vi "Main.vi"(7 "sweep rate, /min":dbl=0.2, 8 "sweep to:":dbl=4.0, 9 "sweep":T8(radio)=enum."2636a_smub") -> ()   [LabVIEW 2021] (continued)
                    n2908 = Concatenate Strings(w3787, w3783, "\t") -> (w3786:string)
                  }
                }
                n2909 = property on="Figure_axis" class="Arr (strict)"("Value"=w3775) -> ()  [unwired: 2 in, 2 out]
                n2910 = property on="data_caption" class="Str"("Value"=w3777) -> ()  [unwired: 2 in, 2 out]
              }
              frame #11 {
                # "2400 1 current measure (2400_1_i)"
                n2911 = local read "2400 1 meas i"() -> (w3794:bool)
                n2912 = property on="Figure_axis" class="Arr (strict)"() -> ("Value"=w3791:string[])  [unwired: 2 in, 2 out]
                n2913 = property on="data_caption" class="Str"() -> ("Value"=w3793:string)  [unwired: 2 in, 2 out]
                n2914 = case shown="False" w3794 {
                  tunnel: w3793 -> [w3796 w3802]
                  tunnel: [w3796 w3801] -> w3792
                  tunnel: w3791 -> [w3795 w3799]
                  tunnel: [w3795 w3797] -> w3790
                  frame False {
                    # "not measure 2400 1 current (2400_1_i)"
                  }
                  frame True {
                    w3798 = "2400_1_i"
                    # "measure 2400 1 current (2400_1_i)"
                    n2915 = local read "2400 1 addr"() -> (w3803:u8)
                    n2916 = Number To Decimal String(number=w3803) -> (decimal integer string=w3804:string)  [unwired: 1 in]
                    n2917 = GPIB Clear(3:w3804) -> ()  [unwired: 1 in, 2 out]
                    n2918 = Build Array (concatenate)(w3799, w3798) -> (w3797:string[])
                    n2919 = Concatenate Strings(w3802, w3798, "\t") -> (w3801:string)
                  }
                }
                n2920 = property on="Figure_axis" class="Arr (strict)"("Value"=w3790) -> ()  [unwired: 2 in, 2 out]
                n2921 = property on="data_caption" class="Str"("Value"=w3792) -> ()  [unwired: 2 in, 2 out]
              }
              frame #12 {
                # "2400 2 voltage measure (2400_2_v)"
                n2922 = local read "2400 2 meas v"() -> (w3809:bool)
                n2923 = property on="Figure_axis" class="Arr (strict)"() -> ("Value"=w3806:string[])  [unwired: 2 in, 2 out]
                n2924 = property on="data_caption" class="Str"() -> ("Value"=w3808:string)  [unwired: 2 in, 2 out]
                n2925 = case shown="False" w3809 {
                  tunnel: w3808 -> [w3811 w3817]
                  tunnel: [w3811 w3816] -> w3807
                  tunnel: w3806 -> [w3810 w3814]
                  tunnel: [w3810 w3812] -> w3805
                  frame False {
                    # "not measure 2400 2 voltage (2400_2_v)"
                  }
                  frame True {
                    w3813 = "2400_2_v"
                    # "measure 2400 2 voltage (2400_2_v)"
                    n2926 = local read "2400 2 addr"() -> (w3818:u8)
                    n2927 = Number To Decimal String(number=w3818) -> (decimal integer string=w3819:string)  [unwired: 1 in]
                    n2928 = GPIB Clear(3:w3819) -> ()  [unwired: 1 in, 2 out]
                    n2929 = Build Array (concatenate)(w3814, w3813) -> (w3812:string[])
                    n2930 = Concatenate Strings(w3817, w3813, "\t") -> (w3816:string)
                  }
                }
                n2931 = property on="Figure_axis" class="Arr (strict)"("Value"=w3805) -> ()  [unwired: 2 in, 2 out]
                n2932 = property on="data_caption" class="Str"("Value"=w3807) -> ()  [unwired: 2 in, 2 out]
              }
              frame #13 {
                # "2400 2 current measure (2400_2_i)"
                n2933 = local read "2400 2 meas i"() -> (w3824:bool)
                n2934 = property on="Figure_axis" class="Arr (strict)"() -> ("Value"=w3821:string[])  [unwired: 2 in, 2 out]
                n2935 = property on="data_caption" class="Str"() -> ("Value"=w3823:string)  [unwired: 2 in, 2 out]
                n2936 = case shown="False" w3824 {
                  tunnel: w3823 -> [w3826 w3832]
                  tunnel: [w3826 w3831] -> w3822
                  tunnel: w3821 -> [w3825 w3829]
                  tunnel: [w3825 w3827] -> w3820
                  frame False {
                    # "not measure 2400 2 current (2400_2_i)"
                  }
                  frame True {
                    w3828 = "2400_2_i"
                    # "measure 2400 2 current (2400_2_i)"
                    n2937 = local read "2400 2 addr"() -> (w3833:u8)
                    n2938 = Number To Decimal String(number=w3833) -> (decimal integer string=w3834:string)  [unwired: 1 in]
                    n2939 = GPIB Clear(3:w3834) -> ()  [unwired: 1 in, 2 out]
                    n2940 = Build Array (concatenate)(w3829, w3828) -> (w3827:string[])
                    n2941 = Concatenate Strings(w3832, w3828, "\t") -> (w3831:string)
                  }
                }
                n2942 = property on="Figure_axis" class="Arr (strict)"("Value"=w3820) -> ()  [unwired: 2 in, 2 out]
                n2943 = property on="data_caption" class="Str"("Value"=w3822) -> ()  [unwired: 2 in, 2 out]
              }
              frame #14 {
                # "2400 3 voltage measure (2400_3_v)"
                n2944 = local read "2400 3 meas v"() -> (w3839:bool)
                n2945 = property on="Figure_axis" class="Arr (strict)"() -> ("Value"=w3836:string[])  [unwired: 2 in, 2 out]
                n2946 = property on="data_caption" class="Str"() -> ("Value"=w3838:string)  [unwired: 2 in, 2 out]
                n2947 = case shown="False" w3839 {
                  tunnel: w3838 -> [w3841 w3847]
                  tunnel: [w3841 w3846] -> w3837
                  tunnel: w3836 -> [w3840 w3844]
                  tunnel: [w3840 w3842] -> w3835
                  frame False {
                    # "not measure 2400 3 voltage (2400_3_v)"
                  }
                  frame True {
                    w3843 = "2400_3_v"
                    # "measure 2400 3 voltage (2400_3_v)"
                    n2948 = local read "2400 3 addr"() -> (w3848:u8)
                    n2949 = Number To Decimal String(number=w3848) -> (decimal integer string=w3849:string)  [unwired: 1 in]
                    n2950 = GPIB Clear(3:w3849) -> ()  [unwired: 1 in, 2 out]
                    n2951 = Build Array (concatenate)(w3844, w3843) -> (w3842:string[])
                    n2952 = Concatenate Strings(w3847, w3843, "\t") -> (w3846:string)
                  }
                }
                n2953 = property on="Figure_axis" class="Arr (strict)"("Value"=w3835) -> ()  [unwired: 2 in, 2 out]
                n2954 = property on="data_caption" class="Str"("Value"=w3837) -> ()  [unwired: 2 in, 2 out]
              }
              frame #15 {
                # "2400 3 current measure (2400_3_i)"
                n2955 = local read "2400 3 meas i"() -> (w3854:bool)
                n2956 = property on="Figure_axis" class="Arr (strict)"() -> ("Value"=w3851:string[])  [unwired: 2 in, 2 out]
                n2957 = property on="data_caption" class="Str"() -> ("Value"=w3853:string)  [unwired: 2 in, 2 out]
                n2958 = case shown="True" w3854 {
                  tunnel: w3853 -> [w3856 w3862]
                  tunnel: [w3856 w3861] -> w3852
                  tunnel: w3851 -> [w3855 w3859]
                  tunnel: [w3855 w3857] -> w3850
                  frame False {
                    # "not measure 2400 3 current (2400_3_i)"
                  }
                  frame True {
                    w3858 = "2400_3_i"
                    # "measure 2400 3 current (2400_3_i)"
                    n2959 = local read "2400 3 addr"() -> (w3863:u8)
                    n2960 = Number To Decimal String(number=w3863) -> (decimal integer string=w3864:string)  [unwired: 1 in]
                    n2961 = GPIB Clear(3:w3864) -> ()  [unwired: 1 in, 2 out]
                    n2962 = Build Array (concatenate)(w3859, w3858) -> (w3857:string[])
                    n2963 = Concatenate Strings(w3862, w3858, "\t") -> (w3861:string)
                  }
                }
                n2964 = property on="Figure_axis" class="Arr (strict)"("Value"=w3850) -> ()  [unwired: 2 in, 2 out]
                n2965 = property on="data_caption" class="Str"("Value"=w3852) -> ()  [unwired: 2 in, 2 out]
              }
              frame #16 {
                # "2182A 1 channel 1 measure (2182A_1_ch1)"
                n2966 = local read "2182A 1 ch1"() -> (w3869:bool)
                n2967 = property on="Figure_axis" class="Arr (strict)"() -> ("Value"=w3866:string[])  [unwired: 2 in, 2 out]
                n2968 = property on="data_caption" class="Str"() -> ("Value"=w3868:string)  [unwired: 2 in, 2 out]
                n2969 = case shown="False" w3869 {
                  tunnel: w3868 -> [w3871 w3877]
                  tunnel: [w3871 w3876] -> w3867
                  tunnel: w3866 -> [w3870 w3874]
                  tunnel: [w3870 w3872] -> w3865
                  frame False {
                    # "not measure 2182A 1 channel 1 (2182A_1_ch1)"
                  }
                  frame True {
                    w3873 = "2182A_1_ch1"
                    # "measure 2182A 1 channel 1 (2182A_1_ch1)"
                    n2970 = local read "2182A 1 addr"() -> (w3878:u8)
                    n2971 = Number To Decimal String(number=w3878) -> (decimal integer string=w3879:string)  [unwired: 1 in]
                    n2972 = GPIB Clear(3:w3879) -> ()  [unwired: 1 in, 2 out]
                    n2973 = Build Array (concatenate)(w3874, w3873) -> (w3872:string[])
                    n2974 = Concatenate Strings(w3877, w3873, "\t") -> (w3876:string)
                  }
                }
                n2975 = property on="Figure_axis" class="Arr (strict)"("Value"=w3865) -> ()  [unwired: 2 in, 2 out]
                n2976 = property on="data_caption" class="Str"("Value"=w3867) -> ()  [unwired: 2 in, 2 out]
              }
              frame #17 {
                # "2182A 1 channel 2 measure (2182A_1_ch2)"
                n2977 = local read "2182A 1 ch2"() -> (w3884:bool)
                n2978 = property on="Figure_axis" class="Arr (strict)"() -> ("Value"=w3881:string[])  [unwired: 2 in, 2 out]
                n2979 = property on="data_caption" class="Str"() -> ("Value"=w3883:string)  [unwired: 2 in, 2 out]
                n2980 = case shown="True" w3884 {
                  tunnel: w3883 -> [w3886 w3892]
                  tunnel: [w3886 w3891] -> w3882
                  tunnel: w3881 -> [w3885 w3889]
                  tunnel: [w3885 w3887] -> w3880
                  frame False {
                    # "not measure 2182A 1 channel 2 (2182A_1_ch2)"
                  }
                  frame True {
                    w3888 = "2182A_1_ch2"
                    # "measure 2182A 1 channel 2 (2182A_1_ch2)"
                    n2981 = local read "2182A 1 addr"() -> (w3893:u8)
                    n2982 = Number To Decimal String(number=w3893) -> (decimal integer string=w3894:string)  [unwired: 1 in]
                    n2983 = GPIB Clear(3:w3894) -> ()  [unwired: 1 in, 2 out]
                    n2984 = Build Array (concatenate)(w3889, w3888) -> (w3887:string[])
                    n2985 = Concatenate Strings(w3892, w3888, "\t") -> (w3891:string)
                  }
                }
                n2986 = property on="Figure_axis" class="Arr (strict)"("Value"=w3880) -> ()  [unwired: 2 in, 2 out]
                n2987 = property on="data_caption" class="Str"("Value"=w3882) -> ()  [unwired: 2 in, 2 out]
              }
              frame #18 {
                # "2182A 2 channel 1 measure (2182A_2_ch1)"
                n2988 = local read "2182A 2 ch1"() -> (w3899:bool)
                n2989 = property on="Figure_axis" class="Arr (strict)"() -> ("Value"=w3896:string[])  [unwired: 2 in, 2 out]
                n2990 = property on="data_caption" class="Str"() -> ("Value"=w3898:string)  [unwired: 2 in, 2 out]
                n2991 = case shown="True" w3899 {
                  tunnel: w3898 -> [w3901 w3907]
                  tunnel: [w3901 w3906] -> w3897
                  tunnel: w3896 -> [w3900 w3904]
                  tunnel: [w3900 w3902] -> w3895
                  frame False {
                    # "not measure 2182A 2 channel 1 (2182A_2_ch1)"
                  }
                  frame True {
                    w3903 = "2182A_2_ch1"
                    # "measure 2182A 2 channel 1 (2182A_2_ch1)"
                    n2992 = local read "2182A 2 addr"() -> (w3908:u8)
                    n2993 = Number To Decimal String(number=w3908) -> (decimal integer string=w3909:string)  [unwired: 1 in]
                    n2994 = GPIB Clear(3:w3909) -> ()  [unwired: 1 in, 2 out]
                    n2995 = Build Array (concatenate)(w3904, w3903) -> (w3902:string[])
                    n2996 = Concatenate Strings(w3907, w3903, "\t") -> (w3906:string)
                  }
                }
                n2997 = property on="Figure_axis" class="Arr (strict)"("Value"=w3895) -> ()  [unwired: 2 in, 2 out]
                n2998 = property on="data_caption" class="Str"("Value"=w3897) -> ()  [unwired: 2 in, 2 out]
              }
              frame #19 {
                # "2182A 2 channel 2 measure (2182A_2_ch2)"
                n2999 = local read "2182A 2 ch2"() -> (w3914:bool)
                n3000 = property on="Figure_axis" class="Arr (strict)"() -> ("Value"=w3911:string[])  [unwired: 2 in, 2 out]
                n3001 = property on="data_caption" class="Str"() -> ("Value"=w3913:string)  [unwired: 2 in, 2 out]
                n3002 = case shown="True" w3914 {
                  tunnel: w3913 -> [w3916 w3922]
                  tunnel: [w3916 w3921] -> w3912
                  tunnel: w3911 -> [w3915 w3919]
                  tunnel: [w3915 w3917] -> w3910
                  frame False {
                    # "not measure 2182A 2 channel 2 (2182A_2_ch2)"
                  }
                  frame True {
                    w3918 = "2182A_2_ch2"
                    # "measure 2182A 2 channel 2 (2182A_2_ch2)"
                    n3003 = local read "2182A 2 addr"() -> (w3923:u8)
                    n3004 = Number To Decimal String(number=w3923) -> (decimal integer string=w3924:string)  [unwired: 1 in]
                    n3005 = GPIB Clear(3:w3924) -> ()  [unwired: 1 in, 2 out]
                    n3006 = Build Array (concatenate)(w3919, w3918) -> (w3917:string[])
                    n3007 = Concatenate Strings(w3922, w3918, "\t") -> (w3921:string)
                  }
                }
                n3008 = property on="Figure_axis" class="Arr (strict)"("Value"=w3910) -> ()  [unwired: 2 in, 2 out]
                n3009 = property on="data_caption" class="Str"("Value"=w3912) -> ()  [unwired: 2 in, 2 out]
              }
              frame #20 {
                # "2182A 3 channel 1 measure (2182A_3_ch1)"
                n3010 = local read "2182A 3 ch1"() -> (w3929:bool)
                n3011 = property on="Figure_axis" class="Arr (strict)"() -> ("Value"=w3926:string[])  [unwired: 2 in, 2 out]
                n3012 = property on="data_caption" class="Str"() -> ("Value"=w3928:string)  [unwired: 2 in, 2 out]
                n3013 = case shown="True" w3929 {
                  tunnel: w3928 -> [w3931 w3937]
                  tunnel: [w3931 w3936] -> w3927
                  tunnel: w3926 -> [w3930 w3934]
                  tunnel: [w3930 w3932] -> w3925
                  frame False {
                    # "not measure 2182A 3 channel 1 (2182A_3_ch1)"
                  }
                  frame True {
                    w3933 = "2182A_3_ch1"
                    # "measure 2182A 3 channel 1 (2182A_3_ch1)"
                    n3014 = local read "2182A 3 addr"() -> (w3938:u8)
                    n3015 = Number To Decimal String(number=w3938) -> (decimal integer string=w3939:string)  [unwired: 1 in]
                    n3016 = GPIB Clear(3:w3939) -> ()  [unwired: 1 in, 2 out]
                    n3017 = Build Array (concatenate)(w3934, w3933) -> (w3932:string[])
                    n3018 = Concatenate Strings(w3937, w3933, "\t") -> (w3936:string)
                  }
                }
                n3019 = property on="Figure_axis" class="Arr (strict)"("Value"=w3925) -> ()  [unwired: 2 in, 2 out]
                n3020 = property on="data_caption" class="Str"("Value"=w3927) -> ()  [unwired: 2 in, 2 out]
              }
              frame #21 {
                # "2182A 3 channel 2 measure (2182A_3_ch2)"
                n3021 = local read "2182A 3 ch2"() -> (w3944:bool)
                n3022 = property on="Figure_axis" class="Arr (strict)"() -> ("Value"=w3941:string[])  [unwired: 2 in, 2 out]
                n3023 = property on="data_caption" class="Str"() -> ("Value"=w3943:string)  [unwired: 2 in, 2 out]
                n3024 = case shown="False" w3944 {
                  tunnel: w3943 -> [w3946 w3952]
                  tunnel: [w3946 w3951] -> w3942
                  tunnel: w3941 -> [w3945 w3949]
                  tunnel: [w3945 w3947] -> w3940
                  frame False {
                    # "not measure 2182A 3 channel 2 (2182A_3_ch2)"
                  }
                  frame True {
                    w3948 = "2182A_3_ch2"
                    # "measure 2182A 3 channel 2 (2182A_3_ch2)"
                    n3025 = local read "2182A 3 addr"() -> (w3953:u8)
                    n3026 = Number To Decimal String(number=w3953) -> (decimal integer string=w3954:string)  [unwired: 1 in]
                    n3027 = GPIB Clear(3:w3954) -> ()  [unwired: 1 in, 2 out]
                    n3028 = Build Array (concatenate)(w3949, w3948) -> (w3947:string[])
                    n3029 = Concatenate Strings(w3952, w3948, "\t") -> (w3951:string)
                  }
                }
                n3030 = property on="Figure_axis" class="Arr (strict)"("Value"=w3940) -> ()  [unwired: 2 in, 2 out]
                n3031 = property on="data_caption" class="Str"("Value"=w3942) -> ()  [unwired: 2 in, 2 out]
              }
              frame #22 {
                # "2182A 4 channel 1 measure (2182A_4_ch1)"
                n3032 = local read "2182A 4 ch1"() -> (w3959:bool)
                n3033 = property on="Figure_axis" class="Arr (strict)"() -> ("Value"=w3956:string[])  [unwired: 2 in, 2 out]
                n3034 = property on="data_caption" class="Str"() -> ("Value"=w3958:string)  [unwired: 2 in, 2 out]
                n3035 = case shown="True" w3959 {
                  tunnel: w3958 -> [w3961 w3967]
                  tunnel: [w3961 w3966] -> w3957
                  tunnel: w3956 -> [w3960 w3964]
                  tunnel: [w3960 w3962] -> w3955
                  frame False {
                    # "not measure 2182A 4 channel 1 (2182A_4_ch1)"
                  }
                  frame True {
                    w3963 = "2182A_4_ch1"
                    # "measure 2182A 4 channel 1 (2182A_4_ch1)"
                    n3036 = local read "2182A 4 addr"() -> (w3968:u8)
                    n3037 = Number To Decimal String(number=w3968) -> (decimal integer string=w3969:string)  [unwired: 1 in]
                    n3038 = GPIB Clear(3:w3969) -> ()  [unwired: 1 in, 2 out]
                    n3039 = Build Array (concatenate)(w3964, w3963) -> (w3962:string[])
                    n3040 = Concatenate Strings(w3967, w3963, "\t") -> (w3966:string)
                  }
                }
                n3041 = property on="Figure_axis" class="Arr (strict)"("Value"=w3955) -> ()  [unwired: 2 in, 2 out]
                n3042 = property on="data_caption" class="Str"("Value"=w3957) -> ()  [unwired: 2 in, 2 out]
              }
              frame #23 {
                # "2182A 4 channel 2 measure (2182A_4_ch2)"
                n3043 = local read "2182A 4 ch2"() -> (w3974:bool)
                n3044 = property on="Figure_axis" class="Arr (strict)"() -> ("Value"=w3971:string[])  [unwired: 2 in, 2 out]
                n3045 = property on="data_caption" class="Str"() -> ("Value"=w3973:string)  [unwired: 2 in, 2 out]
                n3046 = case shown="True" w3974 {
                  tunnel: w3973 -> [w3976 w3982]
                  tunnel: [w3976 w3981] -> w3972
                  tunnel: w3971 -> [w3975 w3979]
                  tunnel: [w3975 w3977] -> w3970
                  frame False {
                    # "not measure 2182A 4 channel 2 (2182A_4_ch2)"
                  }
                  frame True {
                    w3978 = "2182A_4_ch2"
                    # "measure 2182A 4 channel 2 (2182A_4_ch2)"
                    n3047 = local read "2182A 4 addr"() -> (w3983:u8)
                    n3048 = Number To Decimal String(number=w3983) -> (decimal integer string=w3984:string)  [unwired: 1 in]
                    n3049 = GPIB Clear(3:w3984) -> ()  [unwired: 1 in, 2 out]
                    n3050 = Build Array (concatenate)(w3979, w3978) -> (w3977:string[])
                    n3051 = Concatenate Strings(w3982, w3978, "\t") -> (w3981:string)
                  }
                }
                n3052 = property on="Figure_axis" class="Arr (strict)"("Value"=w3970) -> ()  [unwired: 2 in, 2 out]
                n3053 = property on="data_caption" class="Str"("Value"=w3972) -> ()  [unwired: 2 in, 2 out]
              }
              frame #24 {
                # "2636A smua measure voltage (2636A_smua_v)"
                n3054 = local read "2636A smua meas v"() -> (w3989:bool)
                n3055 = property on="Figure_axis" class="Arr (strict)"() -> ("Value"=w3986:string[])  [unwired: 2 in, 2 out]
                n3056 = property on="data_caption" class="Str"() -> ("Value"=w3988:string)  [unwired: 2 in, 2 out]
                n3057 = case shown="True" w3989 {
                  tunnel: w3988 -> [w3991 w4002]
                  tunnel: [w3991 w4001] -> w3987
                  tunnel: w3986 -> [w3990 w3999]
                  tunnel: [w3990 w3997] -> w3985
                  frame False {
                    # "not measure voltage on 2636A smua (2636A_smua_v)"
                  }
                  frame True {
                    w3998 = "2636A_smua_v"
                    # "measure voltage on 2636A smua (2636A_smua_v)"
                    n3058 = local read "2614A addr"() -> (w3993:refnum<visa-resource-name>)
                    n3059 = VISA Open(VISA resource name=w3993) -> (VISA resource name=w3992:refnum<visa-resource-name>, error out=w3994:errorcluster)  [unwired: 4 in]
                    n3060 = VISA Clear(VISA resource name=w3992, error in (no error)=w3994) -> (VISA resource name out=w3996:refnum<visa-resource-name>)  [unwired: 1 out]
                    n3061 = property class="Instr"(reference=w3996, "General Settings:Timeout Value"=u32 10000) -> ()  [unwired: 1 in, 2 out]
                    n3062 = Build Array (concatenate)(w3999, w3998) -> (w3997:string[])
                    n3063 = Concatenate Strings(w4002, w3998, "\t") -> (w4001:string)
                  }
                }
                n3064 = property on="Figure_axis" class="Arr (strict)"("Value"=w3985) -> ()  [unwired: 2 in, 2 out]
                n3065 = property on="data_caption" class="Str"("Value"=w3987) -> ()  [unwired: 2 in, 2 out]
              }
              frame #25 {
                # "2636A smua measure current (2636A_smua_i)"
                n3066 = local read "2636A smua meas i"() -> (w4007:bool)
                n3067 = property on="Figure_axis" class="Arr (strict)"() -> ("Value"=w4004:string[])  [unwired: 2 in, 2 out]
                n3068 = property on="data_caption" class="Str"() -> ("Value"=w4006:string)  [unwired: 2 in, 2 out]
                n3069 = case shown="True" w4007 {
                  tunnel: w4006 -> [w4009 w4020]
                  tunnel: [w4009 w4019] -> w4005
                  tunnel: w4004 -> [w4008 w4017]
                  tunnel: [w4008 w4015] -> w4003
                  frame False {
                    # "not measure current on 2636A smua (2636A_smua_i)"
                  }
                  frame True {
                    w4016 = "2636A_smua_i"
                    # "measure current on 2636A smua (2636A_smua_i)"
                    n3070 = local read "2614A addr"() -> (w4012:refnum<visa-resource-name>)
                    n3071 = VISA Open(VISA resource name=w4012) -> (VISA resource name=w4011:refnum<visa-resource-name>, error out=w4010:errorcluster)  [unwired: 4 in]
                    n3072 = VISA Clear(VISA resource name=w4011, error in (no error)=w4010) -> (VISA resource name out=w4013:refnum<visa-resource-name>)  [unwired: 1 out]
                    n3073 = Build Array (concatenate)(w4017, w4016) -> (w4015:string[])
                    n3074 = property class="Instr"(reference=w4013, "General Settings:Timeout Value"=u32 10000) -> ()  [unwired: 1 in, 2 out]
                    n3075 = Concatenate Strings(w4020, w4016, "\t") -> (w4019:string)
                  }
                }
                n3076 = property on="Figure_axis" class="Arr (strict)"("Value"=w4003) -> ()  [unwired: 2 in, 2 out]
                n3077 = property on="data_caption" class="Str"("Value"=w4005) -> ()  [unwired: 2 in, 2 out]
              }
              frame #26 {
                # "2636A smub measure voltage (2636A_smub_v)"
                n3078 = local read "2636A smub meas v"() -> (w4025:bool)
                n3079 = property on="Figure_axis" class="Arr (strict)"() -> ("Value"=w4022:string[])  [unwired: 2 in, 2 out]
                n3080 = property on="data_caption" class="Str"() -> ("Value"=w4024:string)  [unwired: 2 in, 2 out]
                n3081 = case shown="True" w4025 {
                  tunnel: w4024 -> [w4027 w4038]
                  tunnel: [w4027 w4037] -> w4023
                  tunnel: w4022 -> [w4026 w4035]
                  tunnel: [w4026 w4033] -> w4021
                  frame False {
                    # "not measure voltage on 2636A smub (2636A_smub_v)"
                  }
                  frame True {
                    w4034 = "2636A_smub_v"
                    # "measure voltage on 2636A smub (2636A_smub_v)"
                    n3082 = local read "2614A addr"() -> (w4029:refnum<visa-resource-name>)
                    n3083 = VISA Open(VISA resource name=w4029) -> (VISA resource name=w4028:refnum<visa-resource-name>, error out=w4030:errorcluster)  [unwired: 4 in]
                    n3084 = VISA Clear(VISA resource name=w4028, error in (no error)=w4030) -> (VISA resource name out=w4031:refnum<visa-resource-name>)  [unwired: 1 out]
                    n3085 = Build Array (concatenate)(w4035, w4034) -> (w4033:string[])
                    n3086 = property class="Instr"(reference=w4031, "General Settings:Timeout Value"=u32 10000) -> ()  [unwired: 1 in, 2 out]
                    n3087 = Concatenate Strings(w4038, w4034, "\t") -> (w4037:string)
                  }
                }
                n3088 = property on="Figure_axis" class="Arr (strict)"("Value"=w4021) -> ()  [unwired: 2 in, 2 out]
                n3089 = property on="data_caption" class="Str"("Value"=w4023) -> ()  [unwired: 2 in, 2 out]
              }
              frame #27 {
                # "2636A smub measure current (2636A_smub_i)"
                n3090 = local read "2636A smub meas i"() -> (w4043:bool)
                n3091 = property on="Figure_axis" class="Arr (strict)"() -> ("Value"=w4040:string[])  [unwired: 2 in, 2 out]
                n3092 = property on="data_caption" class="Str"() -> ("Value"=w4042:string)  [unwired: 2 in, 2 out]
                n3093 = case shown="True" w4043 {
                  tunnel: w4042 -> [w4045 w4056]
                  tunnel: [w4045 w4055] -> w4041
                  tunnel: w4040 -> [w4044 w4053]
                  tunnel: [w4044 w4051] -> w4039
                  frame False {
                    # "not measure current on 2636A smub (2636A_smub_i)"
                  }
                  frame True {
                    w4052 = "2636A_smub_i"
                    # "measure current on 2636A smub (2636A_smub_i)"
                    n3094 = local read "2614A addr"() -> (w4046:refnum<visa-resource-name>)
                    n3095 = VISA Open(VISA resource name=w4046) -> (VISA resource name=w4047:refnum<visa-resource-name>, error out=w4048:errorcluster)  [unwired: 4 in]
                    n3096 = VISA Clear(VISA resource name=w4047, error in (no error)=w4048) -> (VISA resource name out=w4049:refnum<visa-resource-name>)  [unwired: 1 out]
                    n3097 = Build Array (concatenate)(w4053, w4052) -> (w4051:string[])
                    n3098 = property class="Instr"(reference=w4049, "General Settings:Timeout Value"=u32 10000) -> ()  [unwired: 1 in, 2 out]
                    n3099 = Concatenate Strings(w4056, w4052, "\t") -> (w4055:string)
                  }
                }
                n3100 = property on="Figure_axis" class="Arr (strict)"("Value"=w4039) -> ()  [unwired: 2 in, 2 out]
                n3101 = property on="data_caption" class="Str"("Value"=w4041) -> ()  [unwired: 2 in, 2 out]
              }
              frame #28 {
                # "measure time"
                n3102 = local read "measure time"() -> (w4061:bool)
                n3103 = property on="Figure_axis" class="Arr (strict)"() -> ("Value"=w4058:string[])  [unwired: 2 in, 2 out]
                n3104 = property on="data_caption" class="Str"() -> ("Value"=w4060:string)  [unwired: 2 in, 2 out]
                n3105 = case shown="True" w4061 {
                  tunnel: w4060 -> [w4063 w4069]
                  tunnel: [w4063 w4068] -> w4059
                  tunnel: w4058 -> [w4062 w4066]
                  tunnel: [w4062 w4064] -> w4057
                  frame False {
                    # "not measuring time"
                  }
                  frame True {
                    w4065 = "time"
                    # "measuring time"
                    n3106 = Build Array (concatenate)(w4066, w4065) -> (w4064:string[])
                    n3107 = Concatenate Strings(w4069, w4065, "\t") -> (w4068:string)
                  }
                }
                n3108 = property on="Figure_axis" class="Arr (strict)"("Value"=w4057) -> ()  [unwired: 2 in, 2 out]
                n3109 = property on="data_caption" class="Str"("Value"=w4059) -> ()  [unwired: 2 in, 2 out]
              }
              frame #29 {
                # "Measure magnetic field on IPS120-0"
                n3110 = local read "MagnetField"() -> (w4074:bool)
                n3111 = property on="Figure_axis" class="Arr (strict)"() -> ("Value"=w4071:string[])  [unwired: 2 in, 2 out]
                n3112 = property on="data_caption" class="Str"() -> ("Value"=w4073:string)  [unwired: 2 in, 2 out]
                n3113 = case shown="True" w4074 {
                  tunnel: w4073 -> [w4076 w4082]
                  tunnel: [w4076 w4081] -> w4072
                  tunnel: w4071 -> [w4075 w4079]
                  tunnel: [w4075 w4077] -> w4070
                  frame False {
                    # "do not Measure magnetic field on IPS120-0"
                  }
                  frame True {
                    w4078 = "MagnetField"
                    n3114 = Build Array (concatenate)(w4079, w4078) -> (w4077:string[])
                    n3115 = Concatenate Strings(w4082, w4078, "\t") -> (w4081:string)
                  }
                }
                n3116 = property on="Figure_axis" class="Arr (strict)"("Value"=w4070) -> ()  [unwired: 2 in, 2 out]
                n3117 = property on="data_caption" class="Str"("Value"=w4072) -> ()  [unwired: 2 in, 2 out]
              }
              frame #30 {
                # "Measure Magnet_T on iPS"
                n3118 = property on="Magnet_T" class="Bool (strict)"() -> ("Value"=w4083:bool)  [unwired: 2 in, 2 out]
                n3119 = property on="Figure_axis" class="Arr (strict)"() -> ("Value"=w4085:string[])  [unwired: 2 in, 2 out]
                n3120 = property on="data_caption" class="Str"() -> ("Value"=w4087:string)  [unwired: 2 in, 2 out]
                n3121 = case shown="True" w4083 {
                  tunnel: w4087 -> [w4089 w4095]
                  tunnel: [w4089 w4094] -> w4086
                  tunnel: w4085 -> [w4088 w4092]
                  tunnel: [w4088 w4090] -> w4084
                  frame False {
                    # "do not Measure magnetic field on IPS120-0"
                  }
                  frame True {
                    w4091 = "Magnet_T"
                    n3122 = Build Array (concatenate)(w4092, w4091) -> (w4090:string[])
                    n3123 = Concatenate Strings(w4095, w4091, "\t") -> (w4094:string)
                  }
                }
                n3124 = property on="Figure_axis" class="Arr (strict)"("Value"=w4084) -> ()  [unwired: 2 in, 2 out]
                n3125 = property on="data_caption" class="Str"("Value"=w4086) -> ()  [unwired: 2 in, 2 out]
              }
              frame #31 {
                # "Measure SH_T on iPS"
                n3126 = property on="PT1" class="Bool (strict)"() -> ("Value"=w4096:bool)  [unwired: 2 in, 2 out]
                n3127 = property on="Figure_axis" class="Arr (strict)"() -> ("Value"=w4098:string[])  [unwired: 2 in, 2 out]
                n3128 = property on="data_caption" class="Str"() -> ("Value"=w4100:string)  [unwired: 2 in, 2 out]
                n3129 = case shown="True" w4096 {
                  tunnel: w4100 -> [w4102 w4108]
                  tunnel: [w4102 w4107] -> w4099
                  tunnel: w4098 -> [w4101 w4105]
                  tunnel: [w4101 w4103] -> w4097
                  frame False {
                    # "do not Measure magnetic field on IPS120-0"
                  }
                  frame True {
                    w4104 = "PT1_Temp"
                    n3130 = Build Array (concatenate)(w4105, w4104) -> (w4103:string[])
                    n3131 = Concatenate Strings(w4108, w4104, "\t") -> (w4107:string)
                  }
                }
                n3132 = property on="Figure_axis" class="Arr (strict)"("Value"=w4097) -> ()  [unwired: 2 in, 2 out]
                n3133 = property on="data_caption" class="Str"("Value"=w4099) -> ()  [unwired: 2 in, 2 out]
              }
              frame #32 {
                # "iTC sample Temp"
                n3134 = property on="MC_RuO2" class="Bool (strict)"() -> ("Value"=w4109:bool)  [unwired: 2 in, 2 out]
                n3135 = property on="Figure_axis" class="Arr (strict)"() -> ("Value"=w4111:string[])  [unwired: 2 in, 2 out]
                n3136 = property on="data_caption" class="Str"() -> ("Value"=w4113:string)  [unwired: 2 in, 2 out]
                n3137 = case shown="True" w4109 {
                  tunnel: w4113 -> [w4115 w4121]
                  tunnel: [w4115 w4120] -> w4112
                  tunnel: w4111 -> [w4114 w4118]
                  tunnel: [w4114 w4116] -> w4110
                  frame False {
                    # "not measure 2461 voltage (2461_meas_v)"
                  }
                  frame True {
                    w4117 = "MC_RuO2_Temp"
                    n3138 = Build Array (concatenate)(w4118, w4117) -> (w4116:string[])
                    n3139 = Concatenate Strings(w4121, w4117, "\t") -> (w4120:string)
                  }
                }
                n3140 = property on="Figure_axis" class="Arr (strict)"("Value"=w4110) -> ()  [unwired: 2 in, 2 out]
                n3141 = property on="data_caption" class="Str"("Value"=w4112) -> ()  [unwired: 2 in, 2 out]
              }
              frame #33 {
                # "iTC sample Temp"
                n3142 = property on="Still" class="Bool (strict)"() -> ("Value"=w4122:bool)  [unwired: 2 in, 2 out]
                n3143 = property on="Figure_axis" class="Arr (strict)"() -> ("Value"=w4124:string[])  [unwired: 2 in, 2 out]
                n3144 = property on="data_caption" class="Str"() -> ("Value"=w4126:string)  [unwired: 2 in, 2 out]
                n3145 = case shown="True" w4122 {
                  tunnel: w4126 -> [w4128 w4134]
                  tunnel: [w4128 w4133] -> w4125
                  tunnel: w4124 -> [w4127 w4131]
                  tunnel: [w4127 w4129] -> w4123
                  frame False {
                    # "not measure 2461 voltage (2461_meas_v)"
                  }
                  frame True {
                    w4130 = "Still_Temp"
                    n3146 = Build Array (concatenate)(w4131, w4130) -> (w4129:string[])
                    n3147 = Concatenate Strings(w4134, w4130, "\t") -> (w4133:string)
                  }
                }
                n3148 = property on="Figure_axis" class="Arr (strict)"("Value"=w4123) -> ()  [unwired: 2 in, 2 out]
                n3149 = property on="data_caption" class="Str"("Value"=w4125) -> ()  [unwired: 2 in, 2 out]
              }
              frame #34 {
                # "iTC sample Temp"
                n3150 = property on="Cold_Plate" class="Bool (strict)"() -> ("Value"=w4135:bool)  [unwired: 2 in, 2 out]
                n3151 = property on="Figure_axis" class="Arr (strict)"() -> ("Value"=w4137:string[])  [unwired: 2 in, 2 out]
                n3152 = property on="data_caption" class="Str"() -> ("Value"=w4139:string)  [unwired: 2 in, 2 out]
                n3153 = case shown="True" w4135 {
                  tunnel: w4139 -> [w4141 w4147]
                  tunnel: [w4141 w4146] -> w4138
                  tunnel: w4137 -> [w4140 w4144]
                  tunnel: [w4140 w4142] -> w4136
                  frame False {
                    # "not measure 2461 voltage (2461_meas_v)"
                  }
                  frame True {
                    w4143 = "Cold_Plate_Temp"
                    n3154 = Build Array (concatenate)(w4144, w4143) -> (w4142:string[])
                    n3155 = Concatenate Strings(w4147, w4143, "\t") -> (w4146:string)
                  }
                }
                n3156 = property on="Figure_axis" class="Arr (strict)"("Value"=w4136) -> ()  [unwired: 2 in, 2 out]
                n3157 = property on="data_caption" class="Str"("Value"=w4138) -> ()  [unwired: 2 in, 2 out]
              }
              frame #35 {
                # "iTC sample Temp"
                n3158 = property on="PT2" class="Bool (strict)"() -> ("Value"=w4148:bool)  [unwired: 2 in, 2 out]
                n3159 = property on="Figure_axis" class="Arr (strict)"() -> ("Value"=w4150:string[])  [unwired: 2 in, 2 out]
                n3160 = property on="data_caption" class="Str"() -> ("Value"=w4152:string)  [unwired: 2 in, 2 out]
                n3161 = case shown="True" w4148 {
                  tunnel: w4152 -> [w4154 w4160]
                  tunnel: [w4154 w4159] -> w4151
                  tunnel: w4150 -> [w4153 w4157]
                  tunnel: [w4153 w4155] -> w4149
                  frame False {
                    # "not measure 2461 voltage (2461_meas_v)"
                  }
                  frame True {
                    w4156 = "PT2_Temp"
                    n3162 = Build Array (concatenate)(w4157, w4156) -> (w4155:string[])
                    n3163 = Concatenate Strings(w4160, w4156, "\t") -> (w4159:string)
                  }
                }
                n3164 = property on="Figure_axis" class="Arr (strict)"("Value"=w4149) -> ()  [unwired: 2 in, 2 out]
                n3165 = property on="data_caption" class="Str"("Value"=w4151) -> ()  [unwired: 2 in, 2 out]
              }
              frame #36 {
                # "iTC sample Temp"
                n3166 = property on="MC_Cernox" class="Bool (strict)"() -> ("Value"=w4161:bool)  [unwired: 2 in, 2 out]
                n3167 = property on="Figure_axis" class="Arr (strict)"() -> ("Value"=w4163:string[])  [unwired: 2 in, 2 out]
                n3168 = property on="data_caption" class="Str"() -> ("Value"=w4165:string)  [unwired: 2 in, 2 out]
                n3169 = case shown="True" w4161 {
                  tunnel: w4165 -> [w4167 w4173]
                  tunnel: [w4167 w4172] -> w4164
                  tunnel: w4163 -> [w4166 w4170]
                  tunnel: [w4166 w4168] -> w4162
                  frame False {
                    # "not measure 2461 voltage (2461_meas_v)"
                  }
                  frame True {
                    w4169 = "MC_Cernox_Temp"
                    n3170 = Build Array (concatenate)(w4170, w4169) -> (w4168:string[])
                    n3171 = Concatenate Strings(w4173, w4169, "\t") -> (w4172:string)
                  }
                }
                n3172 = property on="Figure_axis" class="Arr (strict)"("Value"=w4162) -> ()  [unwired: 2 in, 2 out]
                n3173 = property on="data_caption" class="Str"("Value"=w4164) -> ()  [unwired: 2 in, 2 out]
              }
              frame #37 {
                n3174 = property on="2461_meas_v" class="Bool (strict)"() -> ("Value"=w4174:bool)  [unwired: 2 in, 2 out]
                n3175 = property on="Figure_axis" class="Arr (strict)"() -> ("Value"=w4176:string[])  [unwired: 2 in, 2 out]
                n3176 = property on="data_caption" class="Str"() -> ("Value"=w4178:string)  [unwired: 2 in, 2 out]
                n3177 = case shown="True" w4174 {
                  tunnel: w4178 -> [w4180 w4186]
                  tunnel: [w4180 w4185] -> w4177
                  tunnel: w4176 -> [w4179 w4183]
                  tunnel: [w4179 w4181] -> w4175
                  frame False {
                    # "not measure 2461 voltage (2461_meas_v)"
                  }
                  frame True {
                    w4182 = "2461_meas_v"
                    n3178 = Build Array (concatenate)(w4183, w4182) -> (w4181:string[])
                    n3179 = Concatenate Strings(w4186, w4182, "\t") -> (w4185:string)
                  }
                }
                n3180 = property on="Figure_axis" class="Arr (strict)"("Value"=w4175) -> ()  [unwired: 2 in, 2 out]
                n3181 = property on="data_caption" class="Str"("Value"=w4177) -> ()  [unwired: 2 in, 2 out]
              }
              frame #38 {
                n3182 = property on="2461_meas_i" class="Bool (strict)"() -> ("Value"=w4187:bool)  [unwired: 2 in, 2 out]
                n3183 = property on="Figure_axis" class="Arr (strict)"() -> ("Value"=w4189:string[])  [unwired: 2 in, 2 out]
                n3184 = property on="data_caption" class="Str"() -> ("Value"=w4191:string)  [unwired: 2 in, 2 out]
                n3185 = case shown="True" w4187 {
                  tunnel: w4191 -> [w4193 w4199]
                  tunnel: [w4193 w4198] -> w4190
                  tunnel: w4189 -> [w4192 w4196]
                  tunnel: [w4192 w4194] -> w4188
                  frame False {
                    # "not measure 2461 voltage (2461_meas_v)"
                  }
                  frame True {
                    w4195 = "2461_meas_i"
                    n3186 = Build Array (concatenate)(w4196, w4195) -> (w4194:string[])
                    n3187 = Concatenate Strings(w4199, w4195, "\t") -> (w4198:string)
                  }
                }
                n3188 = property on="Figure_axis" class="Arr (strict)"("Value"=w4188) -> ()  [unwired: 2 in, 2 out]
                n3189 = property on="data_caption" class="Str"("Value"=w4190) -> ()  [unwired: 2 in, 2 out]
              }
              frame #39 {
                # "SR830 1 in phase (SR830_1_ip)"
                n3190 = local read "MFLI1_AuxOut0"() -> (w4204:bool)
                n3191 = property on="Figure_axis" class="Arr (strict)"() -> ("Value"=w4201:string[])  [unwired: 2 in, 2 out]
                n3192 = property on="data_caption" class="Str"() -> ("Value"=w4203:string)  [unwired: 2 in, 2 out]
                n3193 = case shown="True" w4204 {
                  tunnel: w4203 -> [w4206 w4212]
                  tunnel: [w4206 w4211] -> w4202
                  tunnel: w4201 -> [w4205 w4209]
                  tunnel: [w4205 w4207] -> w4200
                  frame False {
                    # "not measure SR830 1 in phase signal (SR830_1_ip)"
                  }
                  frame True {
                    w4208 = "MF1_AuxOut0"
                    n3194 = Build Array (concatenate)(w4209, w4208) -> (w4207:string[])
                    n3195 = Concatenate Strings(w4212, w4208, "\t") -> (w4211:string)
                  }
                }
                n3196 = property on="Figure_axis" class="Arr (strict)"("Value"=w4200) -> ()  [unwired: 2 in, 2 out]
                n3197 = property on="data_caption" class="Str"("Value"=w4202) -> ()  [unwired: 2 in, 2 out]
              }
            }
          }
          frame #2 {
            # "1 = 2400 1\n2 = 2400 2\n3 = 2400 3\n4 = 2636a smua\n5 = 2636a smub\n6 = do not sweep, just time\n7 = Teslatron_iPS_Field\n8 = Teslatron_iTC_Sample T"
            n3198 = property on="sweep" class="RadioBtnsControl (strict)"() -> ("Value"=w4213:T8)  [unwired: 2 in, 2 out]
            n3199 = case "reads current value from instrument which will be sweeping" shown="\"AuxOut0\"" w4213 {
              tunnel: [w4215 w4225 w4234 w4243 w4247 0.0 ("Measuremet") w4253 w4274 w4276 w4281] -> w4214
              frame "2400_1", Default {
                # "reads the voltage on 2400 1"
                n3200 = local read "2400 1 addr"() -> (w4219:u8)
                n3201 = Number To Decimal String(number=w4219) -> (decimal integer string=w4220:string)  [unwired: 1 in]
                n3202 = GPIB Write(0:w4220, 1:":READ?") -> (6:w4216:errorcluster)  [unwired: 3 in, 1 out]
                n3203 = GPIB Read(0:w4220, 1:3200, 3:w4216) -> (5:w4222:string)  [unwired: 2 in, 2 out]
                n3204 = String Subset(string=w4222, length (rest)=13) -> (substring=w4223:string)  [unwired: 1 in]
                n3205 = Fract/Exp String To Number(string=w4223) -> (number=w4215:dbl)  [unwired: 3 in, 1 out]
              }
              frame "2400_2" {
                # "reads the current on 2400 2"
                n3206 = local read "2400 2 addr"() -> (w4229:u8)
                n3207 = Number To Decimal String(number=w4229) -> (decimal integer string=w4230:string)  [unwired: 1 in]
                n3208 = GPIB Write(0:w4230, 1:":READ?") -> (6:w4226:errorcluster)  [unwired: 3 in, 1 out]
                n3209 = GPIB Read(0:w4230, 1:3200, 3:w4226) -> (5:w4232:string)  [unwired: 2 in, 2 out]
                n3210 = String Subset(string=w4232, offset (0)=14, length (rest)=13) -> (substring=w4233:string)
                n3211 = Fract/Exp String To Number(string=w4233) -> (number=w4225:dbl)  [unwired: 3 in, 1 out]
              }
              frame "2400_3" {
                # "reads the voltage on 2400 3"
                n3212 = local read "2400 3 addr"() -> (w4238:u8)
                n3213 = Number To Decimal String(number=w4238) -> (decimal integer string=w4239:string)  [unwired: 1 in]
                n3214 = GPIB Write(0:w4239, 1:":READ?") -> (6:w4235:errorcluster)  [unwired: 3 in, 1 out]
                n3215 = GPIB Read(0:w4239, 1:3200, 3:w4235) -> (5:w4241:string)  [unwired: 2 in, 2 out]
                n3216 = String Subset(string=w4241, length (rest)=13) -> (substring=w4242:string)  [unwired: 1 in]
                n3217 = Fract/Exp String To Number(string=w4242) -> (number=w4234:dbl)  [unwired: 3 in, 1 out]
              }
              frame "2636a_smua" {
                # "reads the voltage on 2636a smua"
                n3218 = local read "2614A addr"() -> (w4246:refnum<visa-resource-name>)
                n3219 = call "SinglePointMeasurement.vi"("Measure"=Measure."Voltage", "Channel"=Channel."a", "VISA resource name 2"=w4246) -> ("Measuremet"=w4243:dbl)  [unwired: 3 in, 4 out]
              }
              frame "2636a_smub" {
                # "reads the voltage on 2636a smub"
                n3220 = local read "2614A addr"() -> (w4250:refnum<visa-resource-name>)
                n3221 = call "SinglePointMeasurement.vi"("Measure"=Measure."Voltage", "Channel"=Channel."b", "VISA resource name 2"=w4250) -> ("Measuremet"=w4247:dbl)  [unwired: 3 in, 4 out]
              }
              frame "time_sweep" {
              }
              frame "iPS" {
                n3222 = property on="Sweep B" class="Bool (strict)"() -> ("Value"=w4252:bool)  [unwired: 2 in, 2 out]
                n3223 = case shown="False" w4252 {
                  tunnel: [w4254 w4272] -> w4253
                  frame False {
                    n3224 = stacked-sequence {
                      tunnel: [_ _ w4261 _] -> w4254
                      frame #0 {
                        n3225 = local read "iPS_addr_sweep"() -> (w4257:refnum<visa-resource-name>)
                        n3226 = property on="sweep to:" class="DigNum (strict)"() -> ("Value"=w4255:dbl)  [unwired: 2 in, 2 out]
                        n3227 = call "iPSset.vi"("Target Field, T"=w4255, "iPSSetCtrl"=iPSsetCtrl."Set Target Field", "VISA resource name"=w4257) -> ()  [unwired: 5 in, 4 out]
                      }
                      frame #1 {
                        n3228 = local read "iPS_addr_sweep"() -> (w4260:refnum<visa-resource-name>)
                        n3229 = property on="sweep rate, /min" class="DigNum (strict)"() -> ("Value"=w4258:dbl)  [unwired: 2 in, 2 out]
                        n3230 = call "iPSset.vi"("Field Rate, T/min"=w4258, "iPSSetCtrl"=iPSsetCtrl."Set Target Field Rate", "VISA resource name"=w4260) -> ()  [unwired: 5 in, 4 out]
                      }
                      frame #2 {
                        n3231 = property on="iPS_addr_sweep" class="VISAName"() -> ("Value"=w4263:refnum<visa-resource-name>)  [unwired: 2 in, 2 out]
                        n3232 = call "iPSread.vi"("iPSreadCtrl"=iPSreadCtrl."OutputField", "VISA resource name"=w4263) -> ("number"=w4261:dbl)  [unwired: 6 in, 3 out]
                      }
                      frame #3 {
                        n3233 = property on="sweep to:" class="DigNum (strict)"() -> ("Value"=w4264:dbl)  [unwired: 2 in, 2 out]
                        n3234 = Not Equal To 0?(x=w4264) -> (x != 0?=w4267:bool)
                        n3235 = local read "iPS_addr_sweep"() -> (w4269:refnum<visa-resource-name>)
                        n3236 = Select(t=iPSsetCtrl."Go to Field" ("iPSSetCtrl"), s=w4267, f=iPSsetCtrl."Go to Field" ("iPSSetCtrl")) -> (s? t:f=w4265:T16)
                        n3237 = call "iPSset.vi"("iPSSetCtrl"=w4265, "VISA resource name"=w4269) -> ()  [unwired: 6 in, 4 out]
                      }
                    }
                  }
                  frame True {
                    # "Measure magnetic field on IPS120-0"
                    n3238 = property on="iPS_addr_sweep" class="VISAName"() -> ("Value"=w4271:refnum<visa-resource-name>)  [unwired: 2 in, 2 out]
                    n3239 = call "iPSread.vi"("iPSreadCtrl"=iPSreadCtrl."OutputField", "VISA resource name"=w4271) -> ("number"=w4272:dbl)  [unwired: 6 in, 3 out]
                  }
                }
              }
              frame "iTC" {
                n3240 = property on="iPS_addr_sweep" class="VISAName"() -> ("Value"=w4273:refnum<visa-resource-name>)  [unwired: 2 in, 2 out]
                n3241 = call "iTCread.vi"("VISA resource name"=w4273, "iTCreadCtrl"=iTCreadCtrl."Sample Temp") -> ("number"=w4274:dbl)  [unwired: 5 in, 3 out]
              }
              frame "2461" {
                n3242 = property on="2461_addr_sweep" class="VISAName"() -> ("Value"=w4277:refnum<visa-resource-name>)  [unwired: 2 in, 2 out]
                n3243 = call <instrlib>:"Get Source Level.vi"("VISA resource name"=w4277) -> ("Current Level Out"=w4276:dbl)  [unwired: 7 in, 3 out]
              }
              frame "AuxOut0" {
                n3244 = property on="MFLI1_addr" class="Str"() -> ("Value"=w4280:string)  [unwired: 2 in, 2 out]
                n3245 = call <instrlib>:"ziOpen.vi"("Address"=w4280) -> ("HandleOut"=w4279:T1)  [unwired: 3 in, 2 out]
                n3246 = call "MFLIcontrol.vi"("MFLI function"=MFLIcommand."Get AuxOut0", "handle in"=w4279) -> ("handle out"=w4278:T1, "AuxOut0_Ampl"=w4281:dbl)  [unwired: 5 in, 3 out]
                n3247 = property on="HandleOut" class="Clust (strict)"("Value"=w4278) -> ()  [unwired: 2 in, 2 out]
              }
            }
          }
          frame #3 {
            # "add \"formula\" string to the axis rings"
            n3248 = property on="Figure_axis" class="Arr (strict)"() -> ("Value"=w4285:string[])  [unwired: 2 in, 2 out]
            n3249 = Build Array (concatenate)(w4285, "formula") -> (w4283:string[])
            n3250 = property on="Figure_axis" class="Arr (strict)"("Value"=w4283) -> ()  [unwired: 2 in, 2 out]
          }
          frame #4 {
            # "passes array to ring"
            n3251 = property on="Figure_axis" class="Arr (strict)"() -> ("Value"=w4287:string[])  [unwired: 2 in, 2 out]
            n3252 = property on="Xaxis" class="Ring (strict)"("Strings []"=w4287) -> ()  [unwired: 2 in, 2 out]
            n3253 = property on="Yright" class="Ring (strict)"("Strings []"=w4287) -> ()  [unwired: 2 in, 2 out]
            n3254 = property on="Yaxis" class="Ring (strict)"("Strings []"=w4287) -> ()  [unwired: 2 in, 2 out]
            n3255 = property on="Stop Ramp" class="Bool"("DisabledEnum"=T10."Enabled" ("Disabled")) -> ()  [unwired: 2 in, 2 out]
          }
        }
        n3256 = call "timeInSeconds.vi"() -> ("Numeric"=w3556:dbl)  [unwired: 2 in, 1 out]
        n3257 = while {
          shift-right: [w4344] -> w3555
          shift-left: w3553 -> [w4343]
          tunnel: w3556 -> [w4341]
          shift-right: [w4335] -> _
          shift-left: w3552 -> [w4336]
          stop <- w4339 stop-if-true
          # "initial value"
          # "this loop stops when target value is reached"
          n3258 = stacked-sequence {
            tunnel: [_ _ w4433 _ _] -> w4338
            tunnel: [_ _ w4432 _ _] -> w4345
            tunnel: w4343 -> [_ _ w4426 _ _]
            tunnel: [w4418 _ _ _ _] -> w4342
            tunnel: w4341 -> [_ _ _ w4454 _]
            tunnel: [_ _ w4426 _ _] -> w4340
            tunnel: [_ _ _ _ w5195] -> w4334
            frame #0 {
              # "time is measured at the beginning\nand at the end of the cycle to\ncalculate delay time required to\nkeep set sweep rate"
              n3259 = flat-sequence {
                tunnel: [w4420] -> w4418
                frame #0 {
                  n3260 = property on="time delay, ms" class="DigNum (strict)"() -> ("Value"=w4419:dbl)  [unwired: 2 in, 2 out]
                  n3261 = Wait (ms)(milliseconds to wait=w4419) -> ()  [unwired: 1 out]
                }
                frame #1 {
                  n3262 = Tick Count (ms)() -> (millisecond timer value=w4420:u32)
                }
              }
            }
            frame #1 {
              w4421 = dbl[] []  # Empty array for data
              # "clear data array before each measurement cycle"
              n3263 = property on="data" class="Arr (strict)"("Value"=w4421) -> ()  [unwired: 2 in, 2 out]
            }
            frame #2 {
              # "add next sweep value to the data array"
              n3264 = property on="Sweep B" class="Bool (strict)"() -> ("Value"=w4423:bool)  [unwired: 2 in, 2 out]
              n3265 = local read "sweep"() -> (w4431:T8)
              n3266 = Not(x=w4423) -> (.not. x?=w4422:bool)
              n3267 = property on="data" class="Arr (strict)"() -> ("Value"=w4428:dbl[])  [unwired: 2 in, 2 out]
              n3268 = Equal?(x=w4431, y=T17."Radio Selection 7" ("sweep")) -> (x = y?=w4425:bool)
              n3269 = And(x=w4425, y=w4422) -> (x .and. y?=w4424:bool)
              n3270 = case shown="True" w4424 {
                tunnel: [w4435 w4452] -> w4433
                tunnel: [w4434 w4451] -> w4432
                tunnel: w4426 -> [_ w4447]
                tunnel: [w4434 w4447] -> w4427
                frame True {
                  # "sweeping magnetic field of Hulk"
                  n3271 = disable-structure shown="Disabled" {
                    frame Disabled {
                      n3272 = stacked-sequence {
                        tunnel: [_ w4443 _] -> _
                        tunnel: [_ _ w4445] -> _
                        frame #0 {
                          n3273 = local read "Hulk_SMS_addr"() -> (w4442:refnum<visa-resource-name>)
                          n3274 = VISA Clear(VISA resource name=w4442) -> ()  [unwired: 1 in, 2 out]
                        }
                        frame #1 {
                          # "acquires current output value"
                          n3275 = local read "Hulk_SMS_addr"() -> (w4444:refnum<visa-resource-name>)
                          n3276 = call "SMS_GET_OUTPUT.vi"("Hulk_SMS_addr"=w4444) -> ("Numeric"=w4443:dbl)  [unwired: 1 in, 2 out]
                        }
                        frame #2 {
                          # "checks, wheter ramp was finished"
                          n3277 = local read "Hulk_SMS_addr"() -> (w4446:refnum<visa-resource-name>)
                          n3278 = call "SMS_RAMP_STATUS.vi"("Hulk_SMS_addr"=w4446) -> ("selection"=w4445:bool)  [unwired: 1 in, 2 out]
                        }
                      }
                    }
                    frame Enabled {
                    }
                  }
                  n3279 = property on="iPS_addr_sweep" class="VISAName"() -> ("Value"=w4438:refnum<visa-resource-name>)  [unwired: 2 in, 2 out]
                  n3280 = property on="sweep to:" class="DigNum (strict)"() -> ("Value"=w4436:dbl)  [unwired: 2 in, 2 out]
                  n3281 = call "iPSread.vi"("iPSreadCtrl"=iPSreadCtrl."MagnetField", "VISA resource name"=w4438) -> ("number"=w4434:dbl)  [unwired: 6 in, 3 out]
                  n3282 = property on="Tolerance_Sweep" class="DigNum (strict)"() -> ("Value"=w4439:dbl)  [unwired: 2 in, 2 out]
                  n3283 = Subtract(x=w4434, y=w4436) -> (x-y=w4441:dbl)
                  n3284 = Absolute Value(x=w4441) -> (abs(x)=w4440:dbl)
                  n3285 = Less Or Equal?(x=w4440, y=w4439) -> (x <= y?=w4435:bool)
                }
                frame False {
                  # "calculate next value"
                  n3286 = property on="sweep to:" class="DigNum (strict)"() -> ("Value"=w4450:dbl)  [unwired: 2 in, 2 out]
                  n3287 = property on="sweep rate, /min" class="DigNum (strict)"() -> ("Value"=w4449:dbl)  [unwired: 2 in, 2 out]
                  n3288 = property on="time/point, sec" class="DigNum (strict)"() -> ("Value"=w4448:dbl)  [unwired: 2 in, 2 out]
                  n3289 = call "CalculateNextValue.vi"("Target a 2"=w4450, "Channel a source value"=w4447, "Ch a sweep rate units/min"=w4449, "time between points, sec"=w4448, "Source a"=Source."Voltage") -> ("Target a"=w4451:dbl, "Boolean"=w4452:bool)
                }
              }
              n3290 = Build Array (concatenate)(w4428, w4427) -> (w4429:dbl[])
              n3291 = property on="data" class="Arr (strict)"("Value"=w4429) -> ()  [unwired: 2 in, 2 out]
            }
            frame #3 {
              n3292 = stacked-sequence "measurement sequence" {
                tunnel: w4454 -> [_ _ _ _ _ _ _ _ _ _ _ _ _ _ _ _ _ _ _ _ _ _ _ _ _ _ _ _ w4854 _ _ _ _ _ _ _ _ _ _ _ _ _ _ _ _ _ _ _ _ _ _ _ _ _ _ _]
                frame #0 {
                  # "check if in-phase\nsignal on lock-in 1 \nis to be measured"
                  n3293 = property on="data" class="Arr (strict)"() -> ("Value"=w4456:dbl[])  [unwired: 2 in, 2 out]
                  n3294 = local read "SR830 1 ip"() -> (w4455:bool)
                  n3295 = case shown="True" w4455 {
                    tunnel: w4456 -> [w4458 w4467]
                    tunnel: [w4458 w4466] -> w4457
                    frame False {
                      # "we are not measuring in phase signal on lock-in 1 (SR830_1_ip)"
                    }
                    frame True {
                      # "we are  measuring lock-in 1, in phase (SR830_1_ip)"
